vi "Delacor_lib_QMH_Enqueue Message (Array).vi"(6 "Priority Message? Array":bool[](array[boolean]), 8 "error in":errorcluster, 9 "Message Data Array":variant[](array[variant]), 10 "Message Array":string[](array[string]), 11 "Message Queue in":refnum<class "ModuleQueue.lvclass">) -> (0 "error out":errorcluster, 3 "Message Queue out":refnum<class "ModuleQueue.lvclass">)   [LabVIEW 2024, in "ModuleQueue.lvclass"]
doc: "For a regular message, enqueue the message. For a priority message, enqueue it at the front of the queue.\nThis is an instance of the polymorphic VI: \"Enqueue Message (poly).vi\"\n____\nDQMH Framework: Palette 7.1.0.1503\nCopyright (c) 2025, DQMH Consortium"
uses:
  ModuleQueue.lvclass
  ModuleQueue.lvclass/ModuleQueue.ctl
  Delacor_lib_QMH_Message--cluster.ctl
panel:
  # "You should not place this polymorphic VI instance directly on your calling code block diagram. \nInstead, you should place 'Enqueue Message (poly).vi' and use the polymorphic selector to choose the desired implementation/type"
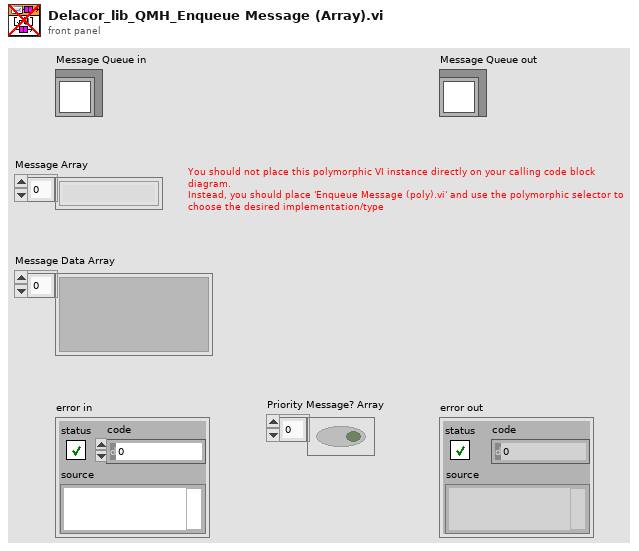
[diagram p1: front panel]
types:
  T1 = typedef "ModuleQueue.lvclass/Delacor_lib_QMH_Message--cluster.ctl" = cluster{"Message":string, "Message Data":variant}
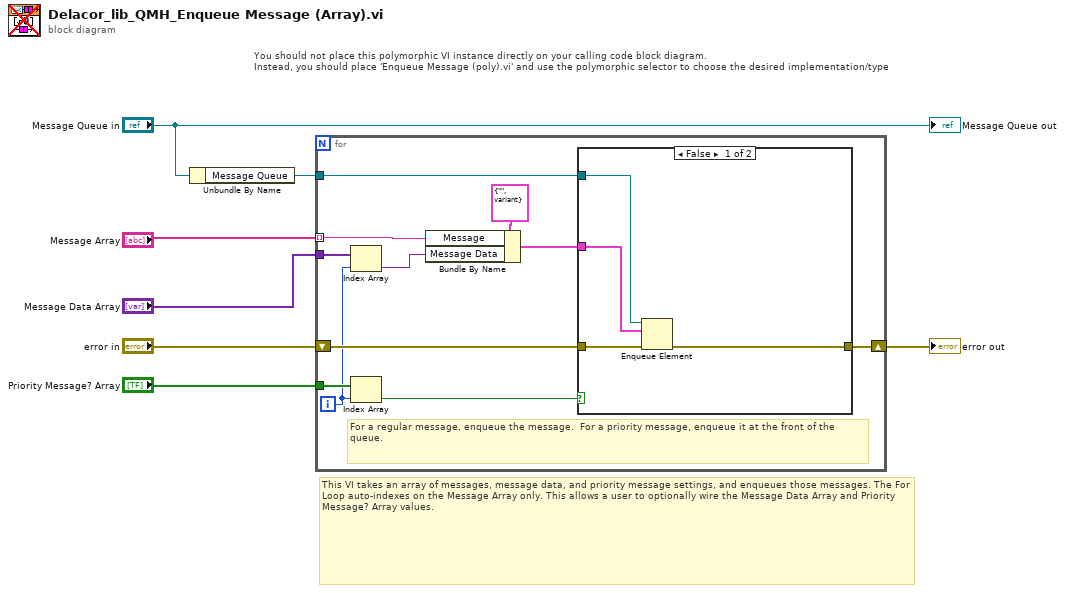
[diagram p0: block diagram]
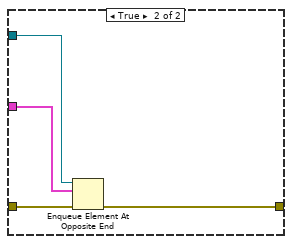
[diagram p2: hidden frame]
diagram:
  # "You should not place this polymorphic VI instance directly on your calling code block diagram. \nInstead, you should place 'Enqueue Message (poly).vi' and use the polymorphic selector to choose the desired implementation/type"
  # "This VI takes an array of messages, message data, and priority message settings, and enqueues those messages. The For Loop auto-indexes on the Message Array only. This allows a user to optionally wire the Message Data Array and Priority Message? Array values."
  n1 = Unbundle By Name("Message Queue in") -> ("Message Queue"=w1:refnum<queue>)
  n2 = for {
    tunnel: "Message Array" -> [w15] mode=indexing
    tunnel: "Message Data Array" -> [w12]
    tunnel: "Priority Message? Array" -> [w10]
    tunnel: w1 -> [w14]
    shift-right: [w17] -> w6
    shift-left: "error in" -> [w18]
    i -> [w8]
    # "For a regular message, enqueue the message.  For a priority message, enqueue it at the front of the queue."
    n3 = Index Array(array=w12, index=w8) -> (element=w11:variant)
    n4 = Index Array(array=w10, index=w8) -> (element=w9:bool)
    n5 = Bundle By Name(cluster=T1 {"Message"="", "Message Data"=variant} ("Message Cluster"), "Message"=w15, "Message Data"=w11) -> (w13:T1)
    n6 = case shown="False" w9 {
      tunnel: w18 -> [w22 w26]
      tunnel: [w21 w25] -> w17
      tunnel: w14 -> [w20 w24]
      tunnel: w13 -> [w19 w23]
      frame False {
        n7 = Enqueue Element(queue=w20, element=w19, error in (no error)=w22) -> (error out=w21:errorcluster)  [unwired: 1 in, 2 out]
      }
      frame True {
        n8 = Enqueue Element At Opposite End(queue=w24, element=w23, error in (no error)=w26) -> (error out=w25:errorcluster)  [unwired: 1 in, 2 out]
      }
    }
  }
  "error out" <- w6
  "Message Queue out" <- "Message Queue in"
